vi "ELVIS III v1.0 DI Block Read.vi"(7 "DI FIFO Sample Rate (Hz)":dbl=1000.0 min=1000.0 max=8000000.0, 8 "error in (no error)":errorcluster, 9 "Number of Samples":u32=1000, 10 "DI (N Samples) Channel List":T3, 11 "myRIO Ref In":T1) -> (0 "error out":errorcluster, 2 "Data by Channel":bool[][](array[boolean]) caption="bool Value List", 3 "myRIO Ref Out":T1)   [LabVIEW 2021]
uses:
  <vilib>/myRIO/Common/Instrument Driver Framework/myRIO v1.0/DI Block/typedefs/DI Block Channels List.ctl
  <vilib>/myRIO/Common/Instrument Driver Framework/myRIO v1.0/DI Block/typedefs/DI Block Channels Enum.ctl
  <vilib>/myRIO/Common/Instrument Driver Framework/Utilities/typedefs/myRIO v1.0 Reference.ctl
  <vilib>/myRIO/Common/Instrument Driver Framework/Utilities/typedefs/Generic FPGA Reference.ctl
  <vilib>/myRIO/Common/Instrument Driver Framework/ELVIS III v1.0/DI Block/typedefs/ELVIS III DI Block FPGA Reference.ctl
  <vilib>/myRIO/Common/Instrument Driver Framework/myRIO v1.0/Resource Manager/vis/myRIO v1.0 Block Write Configuration.vi
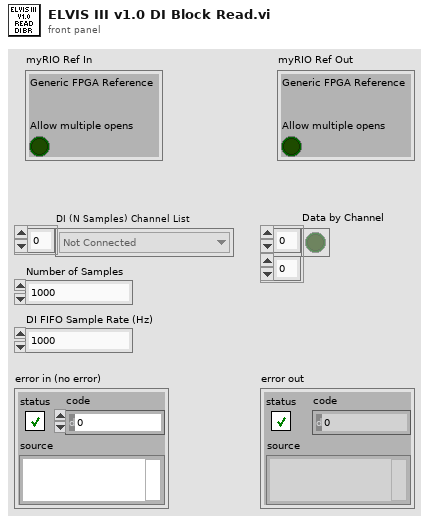
[diagram p1: front panel]
types:
  T1 = typedef "myRIO v1.0 Reference.ctl" = cluster{"Generic FPGA Reference":T2, "Allow multiple opens":bool}
  T2 = typedef "Generic FPGA Reference.ctl" = refnum<k20>
  T3 = typedef "DI Block Channels List.ctl" = T4[]
  T4 = typedef "DI Block Channels Enum.ctl" = enum16{"Not Connected", "A/DI0 (N Samples)", "A/DI1 (N Samples)", "A/DI2 (N Samples)", "A/DI3 (N Samples)", "A/DI4 (N Samples)", "A/DI5 (N Samples)", "A/DI6 (N Samples)", "A/DI7 (N Samples)", "A/DI8 (N Samples)", "A/DI9 (N Samples)", "A/DI10 (N Samples)", "A/DI11 (N Samples)", "A/DI12 (N Samples)", "A/DI13 (N Samples)", "A/DI14 (N Samples)", "A/DI15 (N Samples)", "A/DI16 (N Samples)", "A/DI17 (N Samples)", "A/DI18 (N Samples)", "A/DI19 (N Samples)", "B/DI0 (N Samples)", "B/DI1 (N Samples)", "B/DI2 (N Samples)", "B/DI3 (N Samples)", "B/DI4 (N Samples)", "B/DI5 (N Samples)", "B/DI6 (N Samples)", "B/DI7 (N Samples)", "B/DI8 (N Samples)", "B/DI9 (N Samples)", "B/DI10 (N Samples)", "B/DI11 (N Samples)", "B/DI12 (N Samples)", "B/DI13 (N Samples)", "B/DI14 (N Samples)", "B/DI15 (N Samples)", "B/DI16 (N Samples)", "B/DI17 (N Samples)", "B/DI18 (N Samples)", "B/DI19 (N Samples)"}
  T5 = typedef "ELVIS III DI Block FPGA Reference.ctl" = refnum<k20>
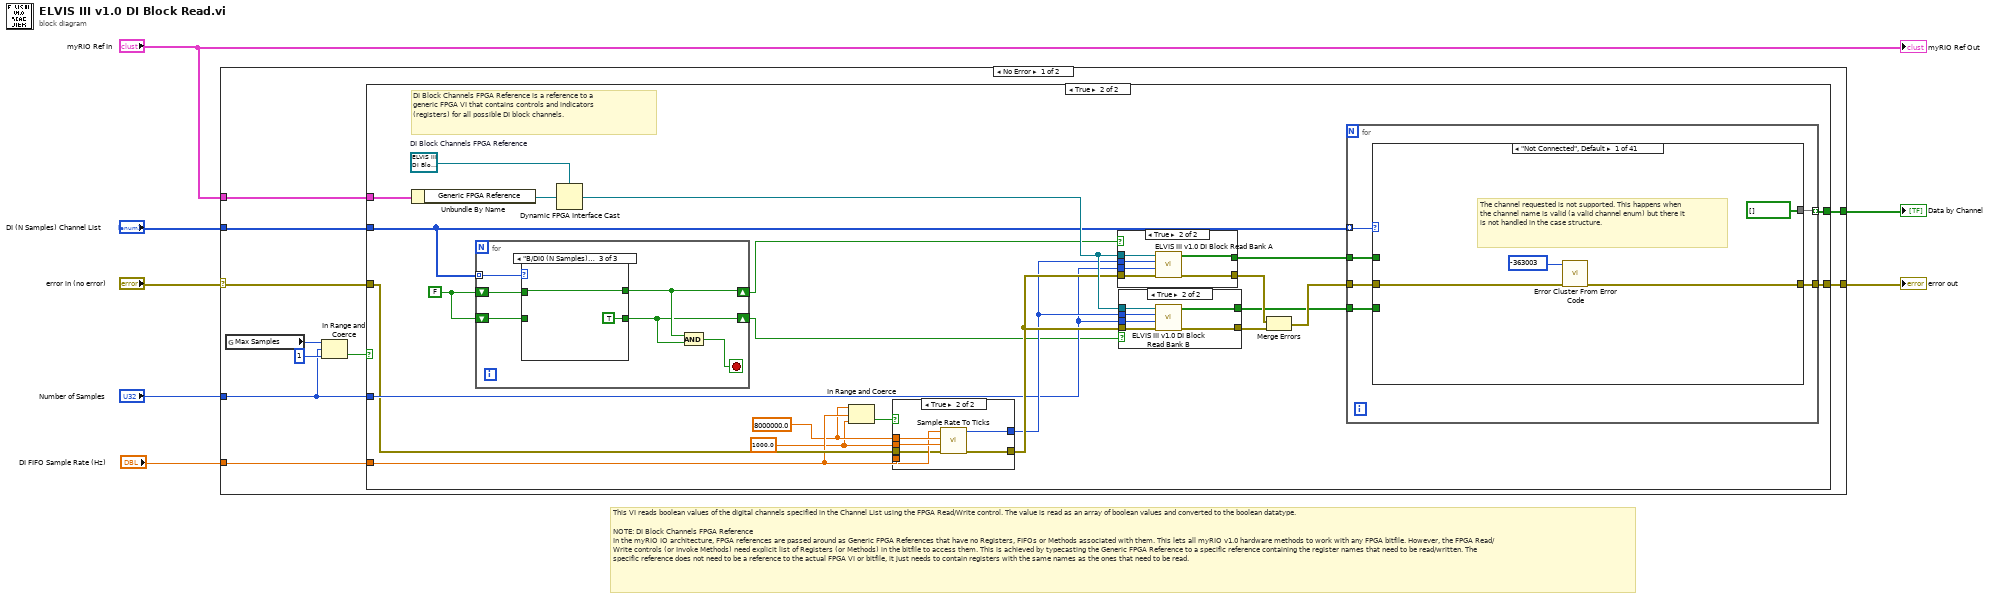
[diagram p0: block diagram]
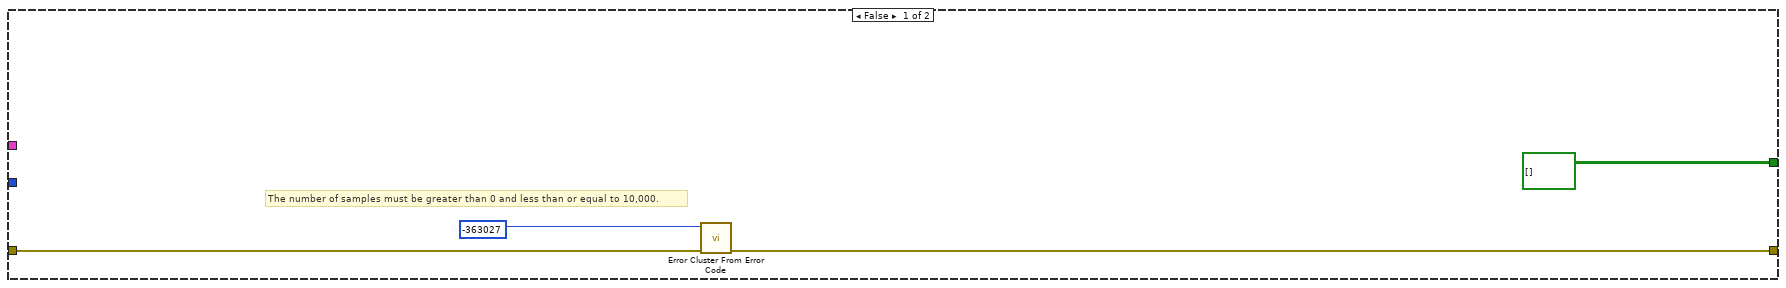
[diagram p2: hidden frame]
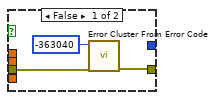
[diagram p3: hidden frame]
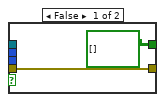
[diagram p4: hidden frame]
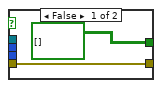
[diagram p5: hidden frame]
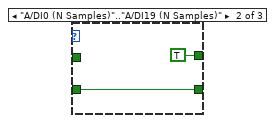
[diagram p7: hidden frame]
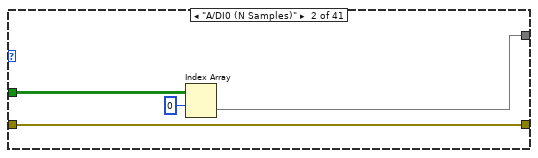
[diagram p8: hidden frame]
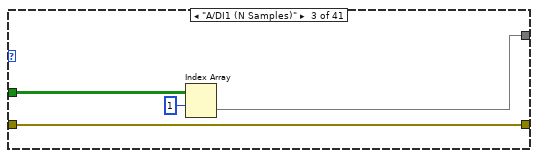
[diagram p9: hidden frame]
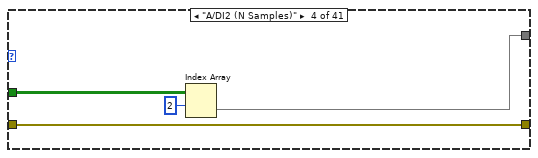
[diagram p10: hidden frame]
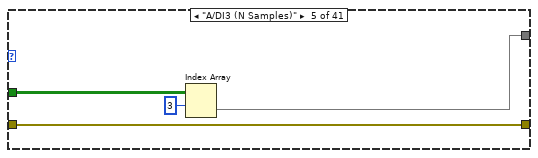
[diagram p11: hidden frame]
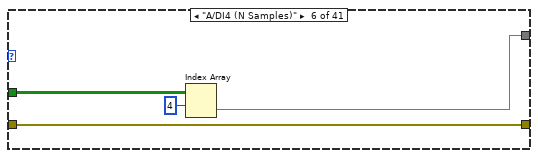
[diagram p12: hidden frame]
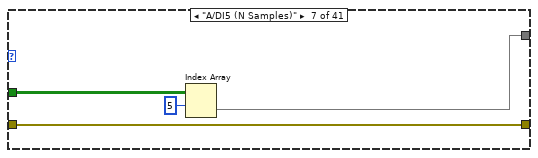
[diagram p13: hidden frame]
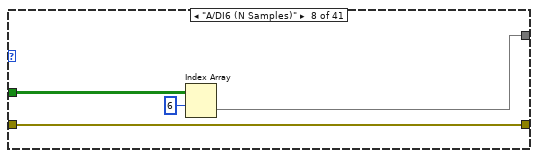
[diagram p14: hidden frame]
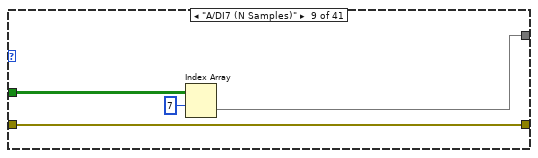
[diagram p15: hidden frame]
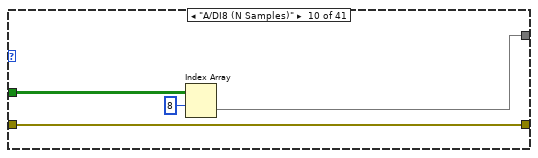
[diagram p16: hidden frame]
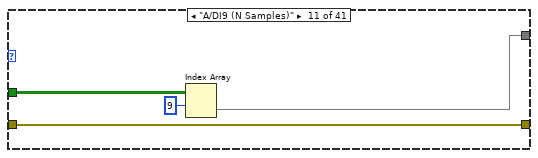
[diagram p17: hidden frame]
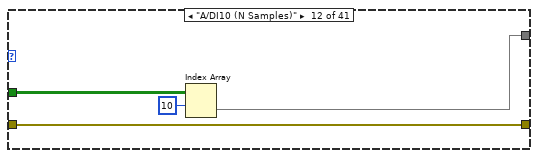
[diagram p18: hidden frame]
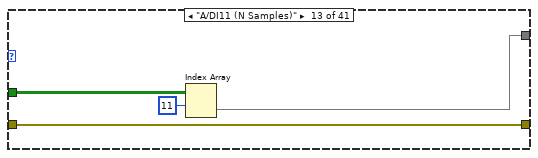
[diagram p19: hidden frame]
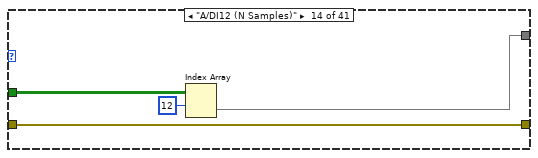
[diagram p20: hidden frame]
diagram:
  # "This VI reads boolean values of the digital channels specified in the Channel List using the FPGA Read/Write control. The value is read as an array of boolean values and converted to the boolean datatype. \n\nNOTE: DI Block Channels FPGA Reference\nIn the myRIO IO architecture, FPGA references are passed around as Generic FPGA References that have no Registers, FIFOs or Methods associated with them. This lets all myRIO v1.0 hardware methods to work with any FPGA bitfile. However, the FPGA Read/Write controls (or Invoke Methods) need explicit list of Registers (or Methods) in the bitfile to access them. This is achieved by typecasting the Generic FPGA Reference to a specific reference containing the register names that need to be read/written. The specific reference does not need to be a reference to the actual FPGA VI or bitfile, it just needs to contain registers with the same names as the ones that need to be read."
  n1 = case shown="No Error" "error in (no error)" {
    selector: "error in (no error)" -> [w12 w253]
    tunnel: "myRIO Ref In" -> [w17 _]
    tunnel: [w15 w253] -> w7
    tunnel: [w16 bool[][] []] -> w5
    tunnel: "DI (N Samples) Channel List" -> [w13 _]
    tunnel: "Number of Samples" -> [w9 _]
    tunnel: "DI FIFO Sample Rate (Hz)" -> [w14 _]
    frame No Error {
      n2 = global read "myRIO v1.0 Block Write Configuration.vi" "Max Samples"() -> (w11:u32)
      n3 = In Range and Coerce(upper limit=w11, x=w9, lower limit=u32 1) -> (In Range?=w8:bool)  [unwired: 1 out]
      n4 = case shown="True" w8 {
        tunnel: w17 -> [_ w43]
        tunnel: [bool[][] [] w41] -> w16
        tunnel: [w19 w40] -> w15
        tunnel: w14 -> [_ w25]
        tunnel: w13 -> [_ w33]
        tunnel: w12 -> [w20 w29]
        tunnel: w9 -> [_ w30]
        frame False {
          # "The number of samples must be greater than 0 and less than or equal to 10,000."
          n5 = call <vilib>:"Error Cluster From Error Code.vi"("error in (no error)"=w20, "error code (0)"=-363027) -> ("error out"=w19:errorcluster)  [unwired: 7 in]
        }
        frame True {
          w28 = FALSE
          w23 = 1000.0
          w24 = 8000000.0
          w44 = T5 refnum  # DI Block Channels FPGA Reference
          # "DI Block Channels FPGA Reference is a reference to a generic FPGA VI that contains controls and indicators (registers) for all possible DI block channels."
          n6 = Unbundle By Name(w43) -> ("Generic FPGA Reference"=w42:T2)
          n7 = for {
            shift-right: [w72] -> w27
            shift-left: w28 -> [w74]
            tunnel: w33 -> [w75] mode=indexing
            shift-right: [w71] -> w26
            shift-left: w28 -> [w73]
            stop <- w70 stop-if-true
            n8 = case shown="\"B/DI0 (N Samples)\"..\"B/DI19 (N Samples)\"" w75 {
              tunnel: [w77 TRUE w81] -> w72
              tunnel: w74 -> [w77 _ w81]
              tunnel: w73 -> [w76 w78 _]
              tunnel: [w76 w78 TRUE] -> w71
              frame "Not Connected", Default {
              }
              frame "A/DI0 (N Samples)".."A/DI19 (N Samples)" {
              }
              frame "B/DI0 (N Samples)".."B/DI19 (N Samples)" {
              }
            }
            n9 = And(x=w72, y=w71) -> (x .and. y?=w70:bool)
          }
          n10 = Dynamic FPGA Interface Cast(Session In=w44, Type=w42) -> (Session Out=w39:T5)
          n11 = In Range and Coerce(upper limit=w24, x=w25, lower limit=w23) -> (In Range?=w22:bool)  [unwired: 1 out]
          n12 = case shown="True" w22 {
            tunnel: w24 -> [_ w53]
            tunnel: w23 -> [_ w52]
            tunnel: w25 -> [_ w51]
            tunnel: [w46 w50] -> w35
            tunnel: [_ w49] -> w34
            tunnel: w29 -> [w45 w48]
            frame False {
              n13 = call <vilib>:"Error Cluster From Error Code.vi"("error in (no error)"=w45, "error code (0)"=-363040) -> ("error out"=w46:errorcluster)  [unwired: 7 in]
            }
            frame True {
              n14 = call <vilib>:"Sample Rate To Ticks.vi"("error in (no error)"=w48, "Minimum (S/s)"=w52, "Maximum (S/s)"=w53, "Sample Rate (S/s)"=w51) -> ("error out"=w50:errorcluster, "Count (tick/s)"=w49:u32)  [unwired: 5 in, 1 out]
            }
          }
          n15 = case shown="True" w27 {
            tunnel: w39 -> [_ w69]
            tunnel: w30 -> [_ w68]
            tunnel: [w63 w67] -> w38
            tunnel: w35 -> [w63 w66]
            tunnel: w34 -> [_ w65]
            tunnel: [bool[][] [] w64] -> w32
            frame False {
            }
            frame True {
              n16 = call <vilib>:"ELVIS III v1.0 DI Block Read Bank A.vi"("error in (no error)"=w66, "Number of Samples"=w68, "Count (tick/s)"=w65, "DI Block Channels FPGA Reference"=w69) -> ("error out"=w67:errorcluster, "Data by Channel"=w64:bool[][])  [unwired: 6 in]
            }
          }
          n17 = case shown="True" w26 {
            tunnel: w39 -> [_ w61]
            tunnel: w30 -> [_ w60]
            tunnel: [w54 w59] -> w37
            tunnel: w35 -> [w54 w58]
            tunnel: w34 -> [_ w57]
            tunnel: [bool[][] [] w56] -> w31
            frame False {
            }
            frame True {
              n18 = call <vilib>:"ELVIS III v1.0 DI Block Read Bank B.vi"("error in (no error)"=w58, "Number of Samples"=w60, "Count (tick/s)"=w57, "DI Block Channels FPGA Reference"=w61) -> ("error out"=w59:errorcluster, "Data by Channel"=w56:bool[][])  [unwired: 6 in]
            }
          }
          n19 = Merge Errors(w38, w37) -> (w36:errorcluster)
          n20 = for {
            tunnel: w33 -> [w84] mode=indexing
            tunnel: w36 -> [w86]
            tunnel: [w87] -> w41 mode=indexing
            tunnel: [w85] -> w40
            tunnel: w32 -> [w83]
            tunnel: w31 -> [w82]
            n21 = case shown="\"Not Connected\", Default" w84 {
              tunnel: [bool[] [] w93 w97 w101 w105 w109 w113 w117 w121 w125 w129 w133 w137 w141 w145 w149 w153 w157 w161 w165 w169 w174 w178 w182 w186 w190 w194 w198 w202 w206 w210 w214 w218 w222 w226 w230 w234 w238 w242 w246 w250] -> w87
              tunnel: w86 -> [w88 w92 w96 w100 w104 w108 w112 w116 w120 w124 w128 w132 w136 w140 w144 w148 w152 w156 w160 w164 w168 w173 w177 w181 w185 w189 w193 w197 w201 w205 w209 w213 w217 w221 w225 w229 w233 w237 w241 w245 w249]
              tunnel: [w89 w92 w96 w100 w104 w108 w112 w116 w120 w124 w128 w132 w136 w140 w144 w148 w152 w156 w160 w164 w168 w173 w177 w181 w185 w189 w193 w197 w201 w205 w209 w213 w217 w221 w225 w229 w233 w237 w241 w245 w249] -> w85
              tunnel: w83 -> [_ w95 w99 w103 w107 w111 w115 w119 w123 w127 w131 w135 w139 w143 w147 w151 w155 w159 w163 w167 w171 _ _ _ _ _ _ _ _ _ _ _ _ _ _ _ _ _ _ _ _]
              tunnel: w82 -> [_ _ _ _ _ _ _ _ _ _ _ _ _ _ _ _ _ _ _ _ _ w172 w176 w180 w184 w188 w192 w196 w200 w204 w208 w212 w216 w220 w224 w228 w232 w236 w240 w244 w248]
              frame "Not Connected", Default {
                # "The channel requested is not supported. This happens when the channel name is valid (a valid channel enum) but there it is not handled in the case structure."
                n22 = call <vilib>:"Error Cluster From Error Code.vi"("error in (no error)"=w88, "error code (0)"=-363003) -> ("error out"=w89:errorcluster)  [unwired: 7 in]
              }
              frame "A/DI0 (N Samples)" {
                n23 = Index Array(array=w95, index (row)=0) -> (element=w93:bool[])  [unwired: 1 in]
              }
              frame "A/DI1 (N Samples)" {
                n24 = Index Array(array=w99, index (row)=1) -> (element=w97:bool[])  [unwired: 1 in]
              }
              frame "A/DI2 (N Samples)" {
                n25 = Index Array(array=w103, index (row)=2) -> (element=w101:bool[])  [unwired: 1 in]
              }
              frame "A/DI3 (N Samples)" {
                n26 = Index Array(array=w107, index (row)=3) -> (element=w105:bool[])  [unwired: 1 in]
              }
              frame "A/DI4 (N Samples)" {
                n27 = Index Array(array=w111, index (row)=4) -> (element=w109:bool[])  [unwired: 1 in]
              }
              frame "A/DI5 (N Samples)" {
                n28 = Index Array(array=w115, index (row)=5) -> (element=w113:bool[])  [unwired: 1 in]
              }
              frame "A/DI6 (N Samples)" {
                n29 = Index Array(array=w119, index (row)=6) -> (element=w117:bool[])  [unwired: 1 in]
              }
              frame "A/DI7 (N Samples)" {
                n30 = Index Array(array=w123, index (row)=7) -> (element=w121:bool[])  [unwired: 1 in]
              }
              frame "A/DI8 (N Samples)" {
                n31 = Index Array(array=w127, index (row)=8) -> (element=w125:bool[])  [unwired: 1 in]
              }
              frame "A/DI9 (N Samples)" {
                n32 = Index Array(array=w131, index (row)=9) -> (element=w129:bool[])  [unwired: 1 in]
              }
              frame "A/DI10 (N Samples)" {
                n33 = Index Array(array=w135, index (row)=10) -> (element=w133:bool[])  [unwired: 1 in]
              }
              frame "A/DI11 (N Samples)" {
                n34 = Index Array(array=w139, index (row)=11) -> (element=w137:bool[])  [unwired: 1 in]
              }
              frame "A/DI12 (N Samples)" {
                n35 = Index Array(array=w143, index (row)=12) -> (element=w141:bool[])  [unwired: 1 in]
              }
              frame "A/DI13 (N Samples)" {
                n36 = Index Array(array=w147, index (row)=13) -> (element=w145:bool[])  [unwired: 1 in]
              }
              frame "A/DI14 (N Samples)" {
                n37 = Index Array(array=w151, index (row)=14) -> (element=w149:bool[])  [unwired: 1 in]
              }
              frame "A/DI15 (N Samples)" {
                n38 = Index Array(array=w155, index (row)=15) -> (element=w153:bool[])  [unwired: 1 in]
              }
              frame "A/DI16 (N Samples)" {
                n39 = Index Array(array=w159, index (row)=16) -> (element=w157:bool[])  [unwired: 1 in]
              }
              frame "A/DI17 (N Samples)" {
                n40 = Index Array(array=w163, index (row)=17) -> (element=w161:bool[])  [unwired: 1 in]
              }
              frame "A/DI18 (N Samples)" {
                n41 = Index Array(array=w167, index (row)=18) -> (element=w165:bool[])  [unwired: 1 in]
              }
              frame "A/DI19 (N Samples)" {
                n42 = Index Array(array=w171, index (row)=19) -> (element=w169:bool[])  [unwired: 1 in]
              }
              frame "B/DI0 (N Samples)" {
                n43 = Index Array(array=w172, index (row)=0) -> (element=w174:bool[])  [unwired: 1 in]
              }
              frame "B/DI1 (N Samples)" {
                n44 = Index Array(array=w176, index (row)=1) -> (element=w178:bool[])  [unwired: 1 in]
              }
              frame "B/DI2 (N Samples)" {
                n45 = Index Array(array=w180, index (row)=2) -> (element=w182:bool[])  [unwired: 1 in]
              }
              frame "B/DI3 (N Samples)" {
                n46 = Index Array(array=w184, index (row)=3) -> (element=w186:bool[])  [unwired: 1 in]
              }
              frame "B/DI4 (N Samples)" {
                n47 = Index Array(array=w188, index (row)=4) -> (element=w190:bool[])  [unwired: 1 in]
              }
              frame "B/DI5 (N Samples)" {
                n48 = Index Array(array=w192, index (row)=5) -> (element=w194:bool[])  [unwired: 1 in]
              }
              frame "B/DI6 (N Samples)" {
                n49 = Index Array(array=w196, index (row)=6) -> (element=w198:bool[])  [unwired: 1 in]
              }
              frame "B/DI7 (N Samples)" {
                n50 = Index Array(array=w200, index (row)=7) -> (element=w202:bool[])  [unwired: 1 in]
              }
              frame "B/DI8 (N Samples)" {
                n51 = Index Array(array=w204, index (row)=8) -> (element=w206:bool[])  [unwired: 1 in]
              }
              frame "B/DI9 (N Samples)" {
                n52 = Index Array(array=w208, index (row)=9) -> (element=w210:bool[])  [unwired: 1 in]
              }
              frame "B/DI10 (N Samples)" {
                n53 = Index Array(array=w212, index (row)=10) -> (element=w214:bool[])  [unwired: 1 in]
              }
              frame "B/DI11 (N Samples)" {
                n54 = Index Array(array=w216, index (row)=11) -> (element=w218:bool[])  [unwired: 1 in]
              }
              frame "B/DI12 (N Samples)" {
                n55 = Index Array(array=w220, index (row)=12) -> (element=w222:bool[])  [unwired: 1 in]
              }
              frame "B/DI13 (N Samples)" {
                n56 = Index Array(array=w224, index (row)=13) -> (element=w226:bool[])  [unwired: 1 in]
              }
              frame "B/DI14 (N Samples)" {
                n57 = Index Array(array=w228, index (row)=14) -> (element=w230:bool[])  [unwired: 1 in]
              }
              frame "B/DI15 (N Samples)" {
                n58 = Index Array(array=w232, index (row)=15) -> (element=w234:bool[])  [unwired: 1 in]
              }
              frame "B/DI16 (N Samples)" {
                n59 = Index Array(array=w236, index (row)=16) -> (element=w238:bool[])  [unwired: 1 in]
              }
              frame "B/DI17 (N Samples)" {
                n60 = Index Array(array=w240, index (row)=17) -> (element=w242:bool[])  [unwired: 1 in]
              }
              frame "B/DI18 (N Samples)" {
                n61 = Index Array(array=w244, index (row)=18) -> (element=w246:bool[])  [unwired: 1 in]
              }
              frame "B/DI19 (N Samples)" {
                n62 = Index Array(array=w248, index (row)=19) -> (element=w250:bool[])  [unwired: 1 in]
              }
            }
          }
        }
      }
    }
    frame Error {
    }
  }
  "error out" <- w7
  "Data by Channel" <- w5
  "myRIO Ref Out" <- "myRIO Ref In"
